vi "LogDebug--callback.vi"(4 "queue out":refnum<queue>, 5 "Event Data":cluster{"sender":refnum<k24>, "e":string}, 6 "Control Ref":refnum<k24>, 7 "Event Common Data":T1) -> ()   [LabVIEW 2025, in "FastTreeView.lvclass"]
uses:
  FastTreeView.lvclass
  FastTreeView.lvclass/FastTreeView.ctl
  C:/Git/FastTreeView/FastTreeView/LV/FastTreeView/dll/FastTreeView.dll
  dll/FastTreeView.dll
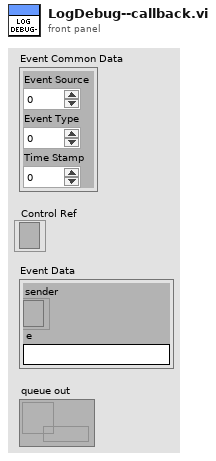
[diagram p1: front panel]
types:
  T1 = cluster{"Event Source":i32, "Event Type":u32, "Time Stamp":u32}
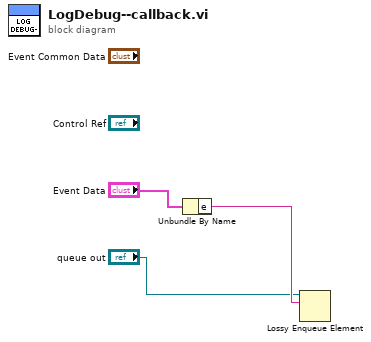
[diagram p0: block diagram]
diagram:
  n1 = Unbundle By Name("Event Data") -> ("e"=w2:string)
  n2 = Lossy Enqueue Element(queue="queue out", element=w2) -> ()  [unwired: 1 in, 4 out]
